vi "Queuing&ADC_test.vi"() -> ()   [LabVIEW 2017]
uses:
  <vilib>/measure/maspectr.llb/Power Spectrum and PSD Export Mode.ctl
  <vilib>/DAQmx/read.llb/DAQmx Read (Analog Wfm 1Chan NSamp).vi
  <vilib>/DAQmx/create/channels.llb/DAQmx Create Channel (AI-Voltage-Basic).vi
  <vilib>/DAQmx/configure/timing.llb/DAQmx Timing (Sample Clock).vi
  <vilib>/DAQmx/miscellaneous.llb/DAQmx Fill In Error Info.vi
  <vilib>/Analysis/3filter.llb/FIR Filter (DBL).vi
  <vilib>/measure/maspectr.llb/FFT Power Spectrum and PSD for 1 Chan.vi
  <vilib>/measure/NI_MAPro.lvlib
  <vilib>/Analysis/NI_AALBase.lvlib
  <vilib>/Analysis/NI_AALPro.lvlib
panel:
  out "RX Signal 5":waveform(dbl)(graph)
  out "RX Signal 4":waveform(dbl)[](graph)
  out "RX Signal 2":waveform(dbl)[](graph)
  in  "Pulse length(sec)":dbl=30000.0 format="%#_6p"
  in  "Frequency2(Hz)":dbl=30000.0 format="%#_6p"
  in  "Frequency1(Hz)":dbl=30000.0 format="%#_6p"
  out "RX Signal 3":cluster{"f0":dbl, "df":dbl, "magnitude":dbl[]}(graph)
  out "RX Signal":waveform(dbl)(graph)
  in  "RX Time(sec)":dbl
  in  "DAQmx 디바이스 이름":tag="PXI2Slot13"
  in  "DAQmx 물리적 채널":tag="PXI2Slot13/ai7"
  in  "sampling rate":dbl=1000.0 caption="속도" format="%0.2f"
  in  "number of sampling":i32=1000 caption="채널당 샘플"
  in  "sample mode":i32(ring)=10123 caption="샘플 모드" items=["유한 샘플"=10178, "연속 샘플"=10123, "하드웨어 타이밍에 의한 단일 포인트"=12522]
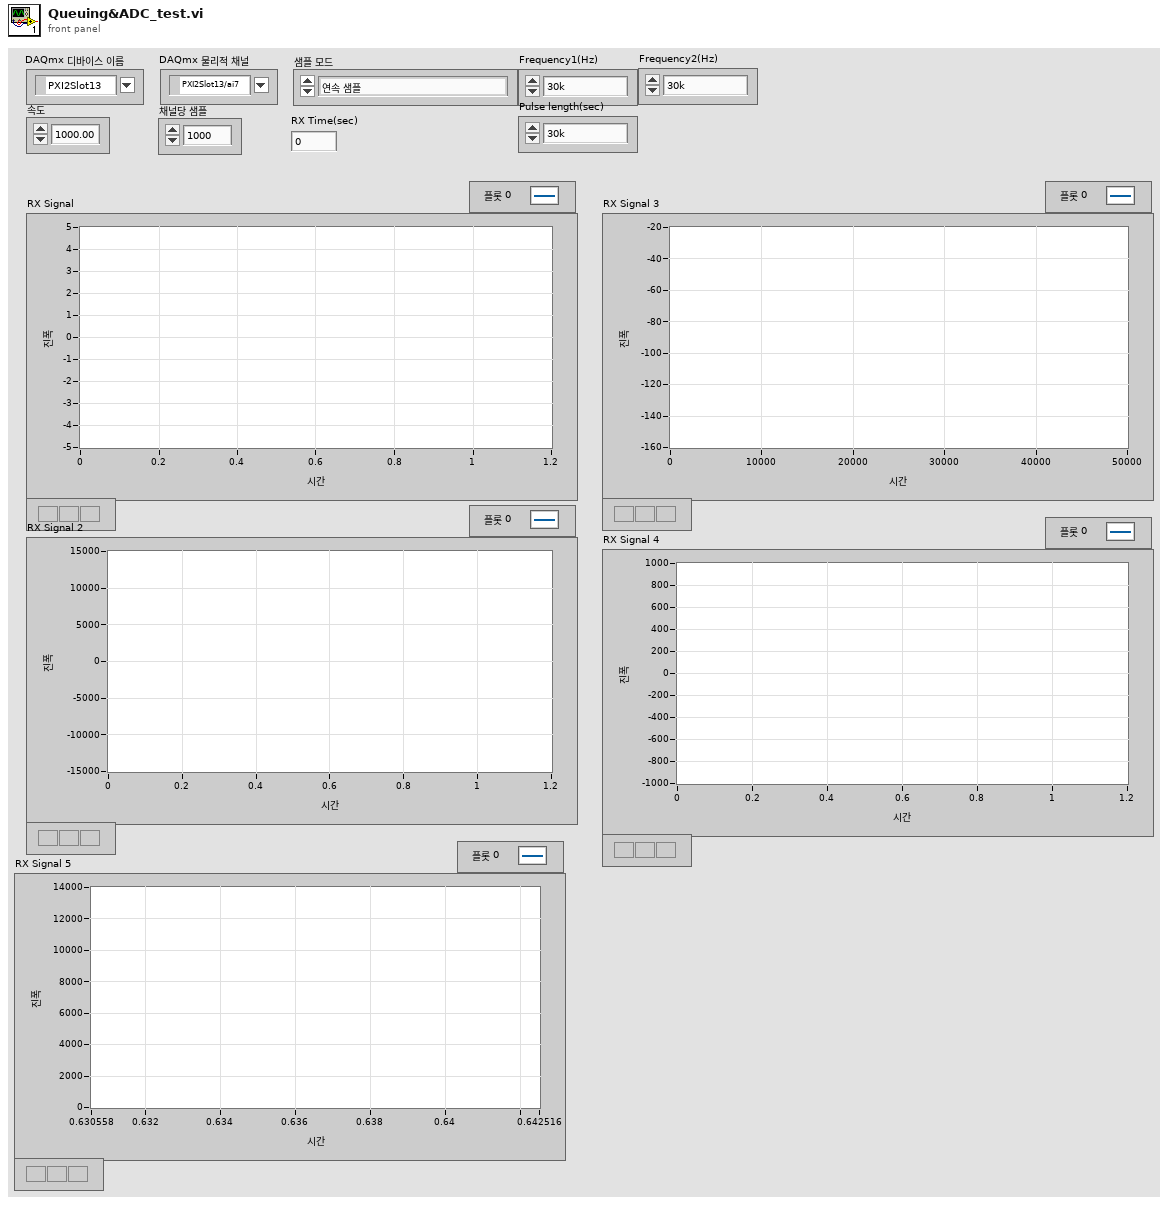
[diagram p1: front panel]
types:
  T1 = typedef "NI_MAPro.lvlib/Power Spectrum and PSD Export Mode.ctl" = u16
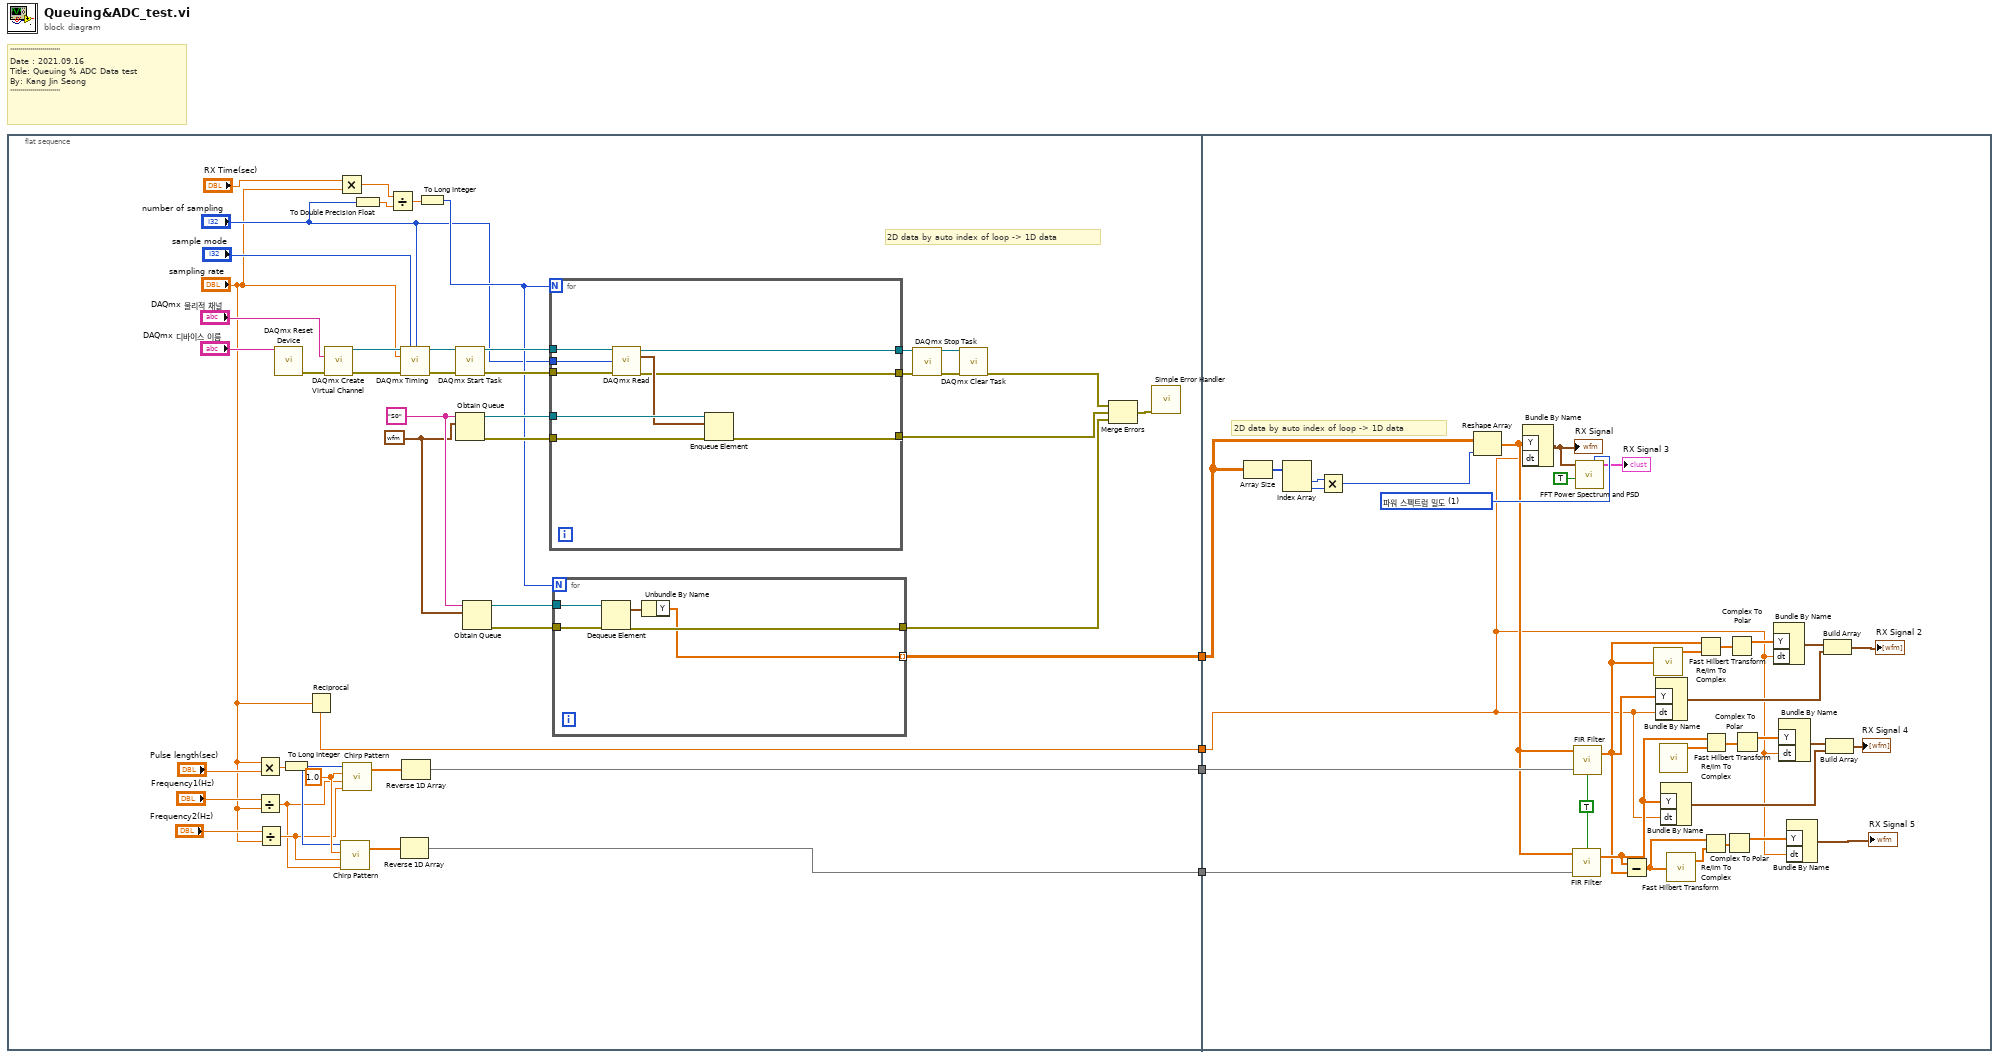
[diagram p0: block diagram]
diagram:
  # "'''''''''''''''''''''''''\nDate : 2021.09.16\nTitle: Queuing % ADC Data test\nBy: Kang Jin Seong\n'''''''''''''''''''''''''"
  n1 = flat-sequence {
    tunnel: [w18] -> w4
    tunnel: [w19] -> w3
    tunnel: [w11] -> w2
    tunnel: [w5] -> w1
    tunnel: w4 -> [w64]
    tunnel: w3 -> [w92]
    tunnel: w2 -> [w87]
    tunnel: w1 -> [w85]
    frame #0 {
      w10 = 1.0 ("amplitude")
      w28 = "S0" ("이름(이름없음)")
      w27 = waveform(dbl) {"t0"=timestamp(0 s since 1904-01-01), "dt"=1.0, "Y"=[]} ("Waveform")
      # "2D data by auto index of loop -> 1D data"
      n2 = Multiply(x="sampling rate", y="Pulse length(sec)") -> (x*y=w16:dbl)
      n3 = Divide(x="Frequency1(Hz)", y="sampling rate") -> (x/y=w7:dbl)
      n4 = Divide(x="Frequency2(Hz)", y="sampling rate") -> (x/y=w8:dbl)
      n5 = call <vilib>:"DAQmx Reset Device.vi"("device in"="DAQmx 디바이스 이름") -> ("error out"=w44:errorcluster)  [unwired: 1 in, 13 out]
      n6 = To Long Integer(number=w16) -> (32bit integer=w9:i32)
      n7 = Reciprocal(x="sampling rate") -> (1/x=w18:dbl)
      n8 = call-poly <vilib>:"DAQmx Create Virtual Channel.vi"("physical channels"="DAQmx 물리적 채널", "error in"=w44) -> ("task out"=w46:refnum<k21>, "error out"=w48:errorcluster)  [unwired: 7 in, 5 out]
      n9 = Multiply(x="RX Time(sec)", y="sampling rate") -> (x*y=w39:dbl)
      n10 = call <vilib>:"Chirp Pattern.vi"("f2"=w7, "f1"=w8, "amplitude"=w10, "samples"=w9) -> ("Chirp Pattern"=w6:dbl[])  [unwired: 1 out]
      n11 = call <vilib>:"Chirp Pattern.vi"("f2"=w8, "f1"=w7, "amplitude"=w10, "samples"=w9) -> ("Chirp Pattern"=w12:dbl[])  [unwired: 1 out]
      n12 = To Double Precision Float(number="number of sampling") -> (double precision float=w38:dbl)
      n13 = Divide(x=w39, y=w38) -> (x/y=w37:dbl)
      n14 = Reverse 1D Array(array=w6) -> (reversed array=w5:dbl[])
      n15 = call-poly <vilib>:"DAQmx Timing.vi"("task/channels in"=w46, "sample mode"="sample mode", "samples per channel"="number of sampling", "rate"="sampling rate", "error in"=w48) -> ("task out"=w49:refnum<k21>, "error out"=w47:errorcluster)  [unwired: 2 in, 7 out]
      n16 = Reverse 1D Array(array=w12) -> (reversed array=w11:dbl[])
      n17 = To Long Integer(number=w37) -> (32bit integer=w21:i32)
      n18 = call <vilib>:"DAQmx Start Task.vi"("task/channels in"=w49, "error in"=w47) -> ("task out"=w32:refnum<k21>, "error out"=w31:errorcluster)  [unwired: 12 in]
      n19 = Obtain Queue(name (unnamed)=w28, element data type=w27) -> (queue out=w36:refnum<queue>, error out=w35:errorcluster)  [unwired: 3 in, 1 out]
      n20 = Obtain Queue(name (unnamed)=w28, element data type=w27) -> (queue out=w26:refnum<queue>, error out=w25:errorcluster)  [unwired: 3 in, 1 out]
      n21 = for {
        N: w21 -> [_]
        tunnel: w36 -> [w63]
        tunnel: w35 -> [w62]
        tunnel: [w61] -> w33
        tunnel: w32 -> [w59]
        tunnel: w31 -> [w58]
        tunnel: [w57] -> w30
        tunnel: [w56] -> w29
        tunnel: "number of sampling" -> [w55]
        n22 = call-poly <vilib>:"DAQmx Read.vi"("task/channels in"=w59, "number of samples per channel"=w55, "error in"=w58) -> ("task out"=w57:refnum<k21>, "data"=w60:waveform(dbl), "error out"=w56:errorcluster)  [unwired: 10 out]
        n23 = Enqueue Element(queue=w63, element=w60, error in (no error)=w62) -> (error out=w61:errorcluster)  [unwired: 1 in, 2 out]
      }
      n24 = for {
        N: w21 -> [_]
        tunnel: w26 -> [w54]
        tunnel: w25 -> [w53]
        tunnel: [w52] -> w24
        tunnel: [w50] -> w19 mode=indexing
        n25 = Dequeue Element(queue=w54, error in (no error)=w53) -> (element=w51:waveform(dbl), error out=w52:errorcluster)  [unwired: 1 in, 2 out]
        n26 = Unbundle By Name(w51) -> ("Y"=w50:dbl[])
      }
      n27 = call <vilib>:"DAQmx Stop Task.vi"("task/channels in"=w30, "error in"=w29) -> ("task out"=w42:refnum<k21>, "error out"=w43:errorcluster)  [unwired: 12 out]
      n28 = call <vilib>:"DAQmx Clear Task.vi"("task in"=w42, "error in"=w43) -> ("error out"=w34:errorcluster)  [unwired: 13 out]
      n29 = Merge Errors(w34, w33, w24) -> (w23:errorcluster)
      n30 = call <vilib>:"Simple Error Handler.vi"("error in (no error)"=w23) -> ()  [unwired: 4 in, 5 out]
    }
    frame #1 {
      w65 = TRUE ("init/cont (init:F)")
      w90 = T1 1 items=["파워 스펙트럼", "파워 스펙트럼 밀도"] ("export mode")
      # "2D data by auto index of loop -> 1D data"
      n31 = Array Size(array=w92) -> (size(s)=w93:i32[])
      n32 = Index Array(array=w93) -> (element #1=w95:i32, element #2=w94:i32)  [unwired: 2 in]
      n33 = Multiply(x=w95, y=w94) -> (x*y=w96:i32)
      n34 = Reshape Array(w92, w96) -> (w86:dbl[])
      n35 = Bundle By Name("Y"=w86, "dt"=w64) -> (w91:waveform(dbl))  [unwired: 1 in]
      "RX Signal" <- w91
      n36 = call-poly <vilib>:"FIR Filter.vi"("init/cont (init:F)"=w65, "FIR Coefficients"=w85, "X"=w86) -> ("Filtered X"=w69:dbl[])  [unwired: 1 in, 1 out]
      n37 = call-poly <vilib>:"FIR Filter.vi"("init/cont (init:F)"=w65, "FIR Coefficients"=w87, "X"=w86) -> ("Filtered X"=w68:dbl[])  [unwired: 1 in, 1 out]
      n38 = call-poly <vilib>:"FFT Power Spectrum and PSD.vi"("export mode"=w90, "dB On (F)"=TRUE, "time signal"=w91) -> ("Power Spectrum / PSD"=→"RX Signal 3":cluster{"f0":dbl, "df":dbl, "magnitude":dbl[]})  [unwired: 5 in, 3 out]
      n39 = Subtract(x=w69, y=w68) -> (x-y=w67:dbl[])
      n40 = call <vilib>:"Fast Hilbert Transform.vi"("X"=w68) -> ("Hilbert{X}"=w84:dbl[])  [unwired: 1 out]
      n41 = Bundle By Name("Y"=w68, "dt"=w64) -> (w80:waveform(dbl))  [unwired: 1 in]
      n42 = call <vilib>:"Fast Hilbert Transform.vi"() -> ("Hilbert{X}"=w78:dbl[])  [unwired: 1 in, 1 out]
      n43 = Bundle By Name("Y"=w69, "dt"=w64) -> (w74:waveform(dbl))  [unwired: 1 in]
      n44 = call <vilib>:"Fast Hilbert Transform.vi"("X"=w67) -> ("Hilbert{X}"=w72:dbl[])  [unwired: 1 out]
      n45 = Re/Im To Complex(1:w84, 2:w68) -> (0:w83:cdb[])
      n46 = Re/Im To Complex(1:w72, 2:w67) -> (0:w71:cdb[])
      n47 = Re/Im To Complex(1:w78, 2:w69) -> (0:w77:cdb[])
      n48 = Complex To Polar(r * e^(i*theta)=w71) -> (r=w70:dbl[])  [unwired: 1 out]
      n49 = Complex To Polar(r * e^(i*theta)=w83) -> (r=w82:dbl[])  [unwired: 1 out]
      n50 = Complex To Polar(r * e^(i*theta)=w77) -> (r=w76:dbl[])  [unwired: 1 out]
      n51 = Bundle By Name("Y"=w82, "dt"=w64) -> (w81:waveform(dbl))  [unwired: 1 in]
      n52 = Bundle By Name("Y"=w76, "dt"=w64) -> (w75:waveform(dbl))  [unwired: 1 in]
      n53 = Bundle By Name("Y"=w70, "dt"=w64) -> (→"RX Signal 5":waveform(dbl))  [unwired: 1 in]
      n54 = Build Array(w81, w80) -> (→"RX Signal 2":waveform(dbl)[])
      n55 = Build Array(w75, w74) -> (→"RX Signal 4":waveform(dbl)[])
    }
  }
